vi "例9.4 连续采集正弦波信号.vi"() -> ()   [LabVIEW 2012]
doc: "本VI说明了从指定设备连续采集声音采样的方式。需要使用连接至声卡的麦克风。可指定需采集的采样数、采样率、通道数和每采样比特率。本VI也将在采样时绘制原始数据。"
uses:
  <vilib>/sound2/lvsound2.llb/Sampling Mode.ctl
  <vilib>/sound2/lvsound2.llb/Sound Input Read (DBL).vi
panel:
  in  "声音格式":cluster{"采样率(S/s)":dbl, "通道数":dbl, "每采样比特数":dbl}={"采样率(S/s)"=44100.0, "通道数"=2.0, "每采样比特数"=16.0}
  out "采集的数据":waveform(dbl)[](graph) caption="采集的波形"
  in  "stop":bool caption="停止"
  in  "Device ID":u32 caption="设备ID" format="%.0x"
  in  "Number of Samples/ch":i32=5000 caption="每通道采样数"
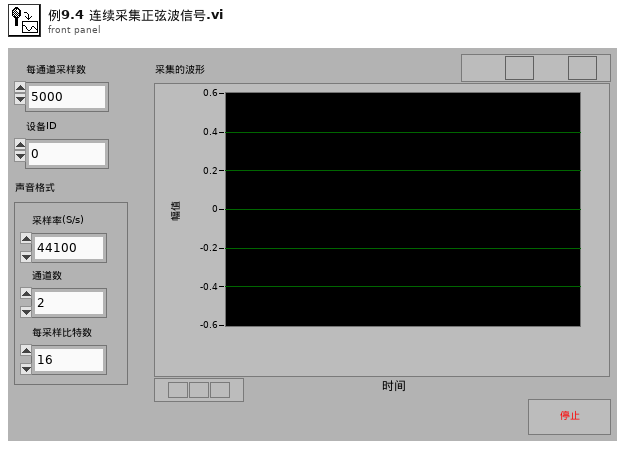
[diagram p1: front panel]
types:
  T1 = typedef "Sampling Mode.ctl" = i32
  T2 = typedef "Sound Input Task ID.ctl" = u32
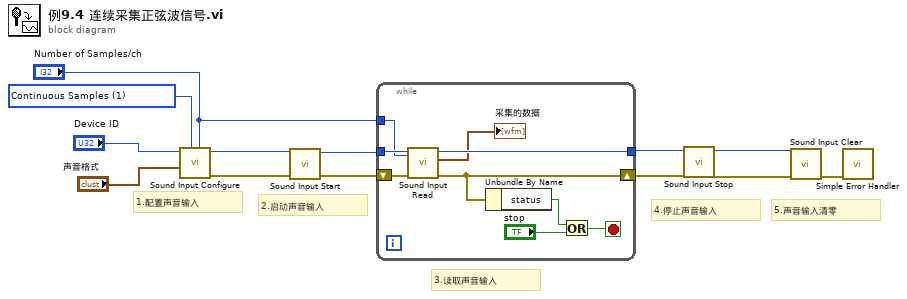
[diagram p0: block diagram]
diagram:
  w12 = T1 1 items=["Finite Samples", "Continuous Samples"] ("sample mode")
  # "5.声音输入清零"
  # "4.停止声音输入"
  # "3.读取声音输入"
  # "2.启动声音输入"
  # "1.配置声音输入"
  n1 = call <vilib>:"Sound Input Configure.vi"("number of samples/ch"="Number of Samples/ch", "sample mode"=w12, "sound format"="声音格式", "device ID"="Device ID") -> ("error out"=w5:errorcluster, "task ID"=w8:T2)  [unwired: 6 in]
  n2 = call <vilib>:"Sound Input Start.vi"("error in (no error)"=w5, "task ID"=w8) -> ("error out"=w6:errorcluster, "task ID out"=w7:T2)  [unwired: 8 in]
  n3 = while {
    tunnel: w7 -> [w21]
    tunnel: [w20] -> w4
    tunnel: "Number of Samples/ch" -> [w15]
    shift-right: [w16] -> w3
    shift-left: w6 -> [w22]
    stop <- w17 stop-if-true
    n4 = call-poly <vilib>:"Sound Input Read.vi"("number of samples/ch"=w15, "error in (no error)"=w22, "task ID"=w21) -> ("error out"=w16:errorcluster, "data"=→"采集的数据":waveform(dbl)[], "task ID out"=w20:T2)  [unwired: 6 in]
    n5 = Unbundle By Name(w16) -> ("status"=w19:bool)
    n6 = Or(x=w19, y="stop") -> (x .or. y?=w17:bool)
  }
  n7 = call <vilib>:"Sound Input Stop.vi"("error in (no error)"=w3, "task ID"=w4) -> ("error out"=w1:errorcluster, "task ID out"=w2:T2)  [unwired: 8 in]
  n8 = call <vilib>:"Sound Input Clear.vi"("error in (no error)"=w1, "task ID"=w2) -> ("error out"=w10:errorcluster)  [unwired: 9 in]
  n9 = call <vilib>:"Simple Error Handler.vi"("error in (no error)"=w10) -> ()  [unwired: 4 in, 5 out]
